vi "ThermocoupleLog.vi"() -> ()   [LabVIEW 2024]
uses:
  <vilib>/Instr/_visa.llb/VISA Configure Serial Port (Instr).vi
panel:
  out "Waveform Chart":dbl(graph)
  out "appended array":dbl[](array[numeric])
  out "error out":errorcluster
  in  "stop":bool
  # "Thermocouple (C)"
  # "Ambient (C)"
  # "Delta (C)"
  # "Time (s)"
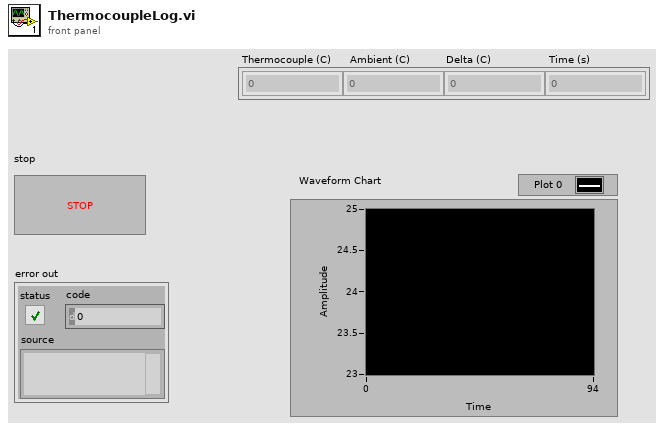
[diagram p1: front panel]
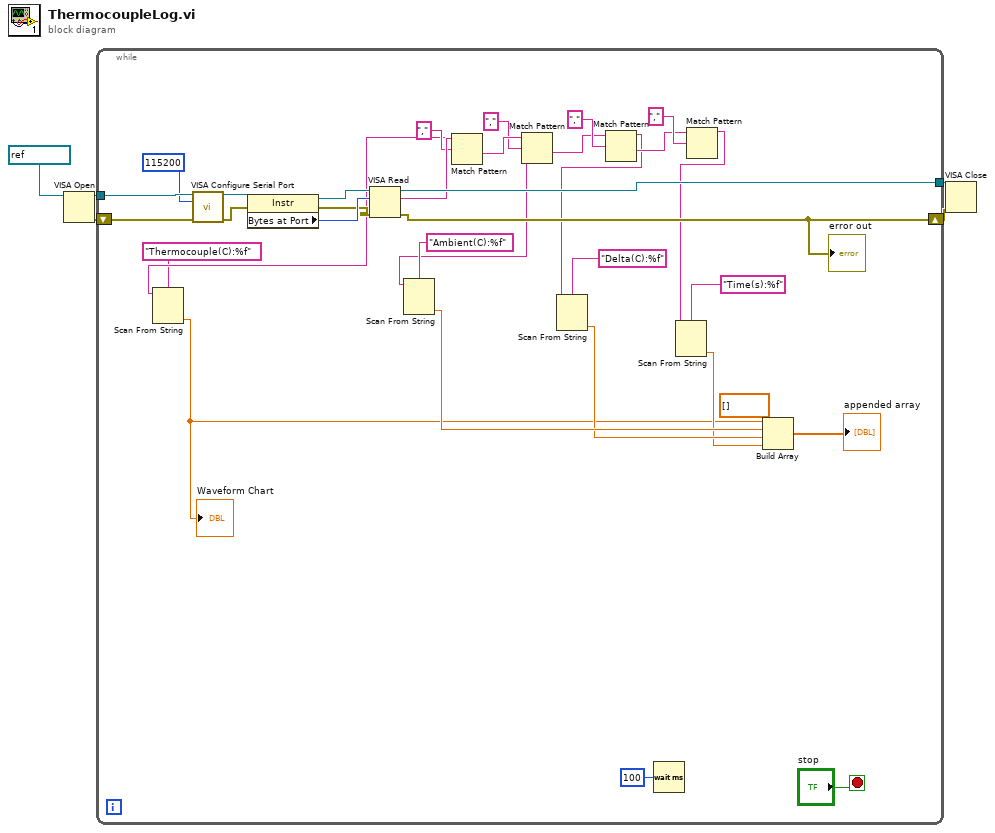
[diagram p0: block diagram]
diagram:
  n1 = VISA Open(VISA resource name=refnum<visa-resource-name> "COM4") -> (VISA resource name=w4:refnum<visa-resource-name>, error out=w3:errorcluster)  [unwired: 4 in]
  n2 = while {
    tunnel: w4 -> [w35]
    tunnel: [w36] -> w2
    shift-right: [w17] -> w1
    shift-left: w3 -> [w33]
    stop <- "stop" stop-if-true
    (unwired) dbl[] [] ("appended array")
    n3 = call-poly "VISA Configure Serial Port"("VISA resource name"=w35, "baud rate (9600)"=u32 115200, "error in (no error)"=w33) -> ("VISA resource name out"=w32:refnum<visa-resource-name>, "error out"=w29:errorcluster)  [unwired: 11 in]
    n4 = property class="Instr"(reference=w32, error in=w29) -> (reference out=w27:refnum<visa-resource-name>, error out=w26:errorcluster, "Bytes at Port"=w28:u32)
    n5 = VISA Read(VISA resource name=w27, byte count=w28, error in (no error)=w26) -> (VISA resource name out=w36:refnum<visa-resource-name>, read buffer=w31:string, error out=w17:errorcluster)  [unwired: 1 out]
    "error out" <- w17
    n6 = Match Pattern(string=w31, regular expression=",") -> (before substring=w19:string, after substring=w25:string)  [unwired: 1 in, 2 out]
    n7 = Scan From String(format string="Thermocouple(C):%f", input string=w19) -> (output 1=w6:dbl)  [unwired: 3 in, 3 out]
    "Waveform Chart" <- w6
    n8 = Match Pattern(string=w25, regular expression=",") -> (before substring=w15:string, after substring=w22:string)  [unwired: 1 in, 2 out]
    n9 = Scan From String(format string="Ambient(C):%f", input string=w15) -> (output 1=w10:dbl)  [unwired: 3 in, 3 out]
    n10 = Match Pattern(string=w22, regular expression=",") -> (before substring=w13:string, after substring=w20:string)  [unwired: 1 in, 2 out]
    n11 = Scan From String(format string="Delta(C):%f", input string=w13) -> (output 1=w9:dbl)  [unwired: 3 in, 3 out]
    n12 = Wait (ms)(milliseconds to wait=u32 100) -> ()  [unwired: 1 out]
    n13 = Match Pattern(string=w20, regular expression=",") -> (before substring=w11:string)  [unwired: 1 in, 3 out]
    n14 = Scan From String(format string="Time(s):%f", input string=w11) -> (output 1=w8:dbl)  [unwired: 3 in, 3 out]
    n15 = Build Array(w6, w10, w9, w8) -> (→"appended array":dbl[])
  }
  n16 = VISA Close(VISA resource name=w2, error in (no error)=w1) -> ()  [unwired: 1 out]
